vi "Ball Loading Screen.vi"(8 "Cluster width":i32=200, 9 "Main Loop Iterations":i32=5, 10 "Ball Refs":refnum<vi>[](array[refnum]), 11 "Positions In":i32[](array[numeric])) -> (3 "Positions Out":i32[](array[numeric]))   [LabVIEW 2014, in "Endigit.lvlib"]
uses:
  Endigit.lvlib
panel:
  # "https://decibel.ni.com/content/docs/DOC-1086"
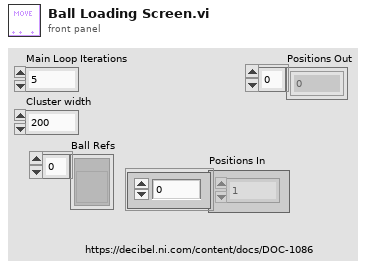
[diagram p1: front panel]
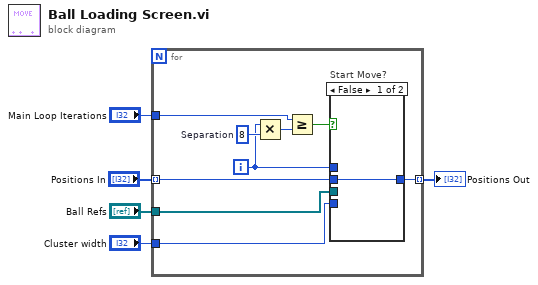
[diagram p0: block diagram]
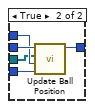
[diagram p2: hidden frame]
diagram:
  n1 = for {
    tunnel: [w14] -> w5 mode=indexing
    tunnel: "Positions In" -> [w13] mode=indexing
    tunnel: "Ball Refs" -> [w11]
    tunnel: "Main Loop Iterations" -> [w8]
    tunnel: "Cluster width" -> [w6]
    i -> [w10]
    w12 = 8  # Separation
    n2 = Multiply(x=w10, y=w12) -> (x*y=w9:i32)
    n3 = Greater Or Equal?(x=w8, y=w9) -> (x >= y?=w7:bool)
    n4 = case "Start Move?" shown="False" w7 {
      tunnel: [w15 w20] -> w14
      tunnel: w13 -> [w15 w19]
      tunnel: w10 -> [_ w18]
      tunnel: w11 -> [_ w17]
      tunnel: w6 -> [_ w16]
      frame False {
      }
      frame True {
        n5 = call "Update Ball Position.vi"("Cluster width"=w16, "Ball Nr"=w18, "Ball Refs"=w17, "Position In"=w19) -> ("Position out"=w20:i32)  [unwired: 7 in]
      }
    }
  }
  "Positions Out" <- w5
